vi "Set Image.vi"(5 "vend":i32, 6 "vstart":i32, 7 "hend":i32, 9 "hstart":i32, 10 "vbin":i32, 11 "hbin":i32) -> (3 "function return":u32)   [LabVIEW 2018, in "Copy of Andor SDK.lvlib"]
doc: "EXPNETTYPE unsigned int WINAPI SetImage(int hbin, int vbin, int hstart, int hend, int vstart, int vend);"
uses:
  Copy of Andor SDK.lvlib
  <userlib>/Andor SDK/ATMCD32D.dll
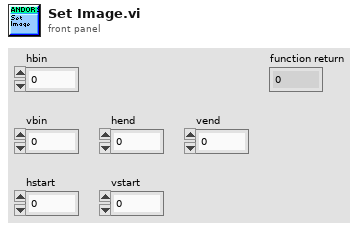
[diagram p1: front panel]
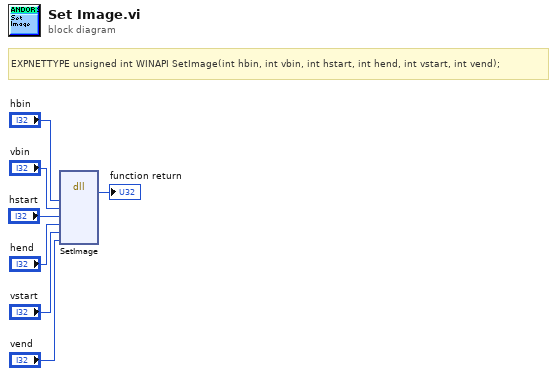
[diagram p0: block diagram]
diagram:
  # "EXPNETTYPE unsigned int WINAPI SetImage(int hbin, int vbin, int hstart, int hend, int vstart, int vend);"
  n1 = dll-call lib="C:/Program Files (x86)/National Instruments/LabVIEW 2018/user.lib/Andor SDK/ATMCD32D.*" fn="SetImage"("hbin"="hbin", "vbin"="vbin", "hstart"="hstart", "hend"="hend", "vstart"="vstart", "vend"="vend") -> (→"function return":u32)  [unwired: 9 in, 2 out]
